vi "CLC_GEN3_L2_InPhaseCal_mW.vi"() -> ()   [LabVIEW 2023, in "Clover_Cell.lvlib"]
uses:
  Clover_Cell.lvlib
  lib/Anritsu Signal Analyzer Series/Anritsu Signal Analyzer Series.lvlib
  lib/ELTA/ELTA.lvlib
panel:
  in  "Daul_Ch_Phase_Sweep":bool
  in  "SweepSwitch?":u16(ring) items=["NoSweep(Single)", "Sweep"]
  in  "SweepMode":u16(ring) items=["Phase", "Gain"]
  in  "Method":u16(ring)=1 items=["dBm"=1, "mW"=2]
  in  "Polarity":u16(ring) items=["H", "V"]
  in  "VISA resource name":refnum<visa-resource-name>="TCPIP0::192.168.100.230::inst0::INSTR"
  in  "CenterFreq(GHz)":dbl=28.0
  in  "AvgTimes":i32=3
  in  "Single_Ch_Phase_Sweep":bool
  in  "TRXmode":u16(ring)=1 items=["Rx"=2, "Tx"=1]
  out "GainStep":i32=63
  out "PhaseStep":i32=63
  out "Channel":i32=63
  out "Total mW":dbl format="%.7f"
  out "Total dBm":dbl format="%.7f"
  out "Ref. mW":dbl format="%.7f"
  out "Ref. dBm":dbl format="%.7f"
  out "Main mW":dbl format="%.7f"
  out "Main dBm":dbl format="%.7f"
  out "Data":dbl[][](array[numeric])
  out "FileNAME_Single":string
  out "Spectrum Analyzer":dbl[](graph)
  out "CurrentData":dbl[](array[numeric])
  out "Duration":dbl
  out "TotalTime":dbl format="%.2f"
  out "StopTime":timestamp=timestamp(3663835912.033212 s since 1904-01-01)
  out "FileNAME_Dual":string
  out "StartTime":timestamp=timestamp(3663835741.875155 s since 1904-01-01)
  out "TX/RX":u16=1
  out "error out":errorcluster
  out "output cluster":T1={"address"="192.168.100.111", "remote port or service name"=5025, "timeout ms (60000)"=10000}
  out "Operating \nChannel(s)":bool[][](array[boolean])
  out "OK?":bool
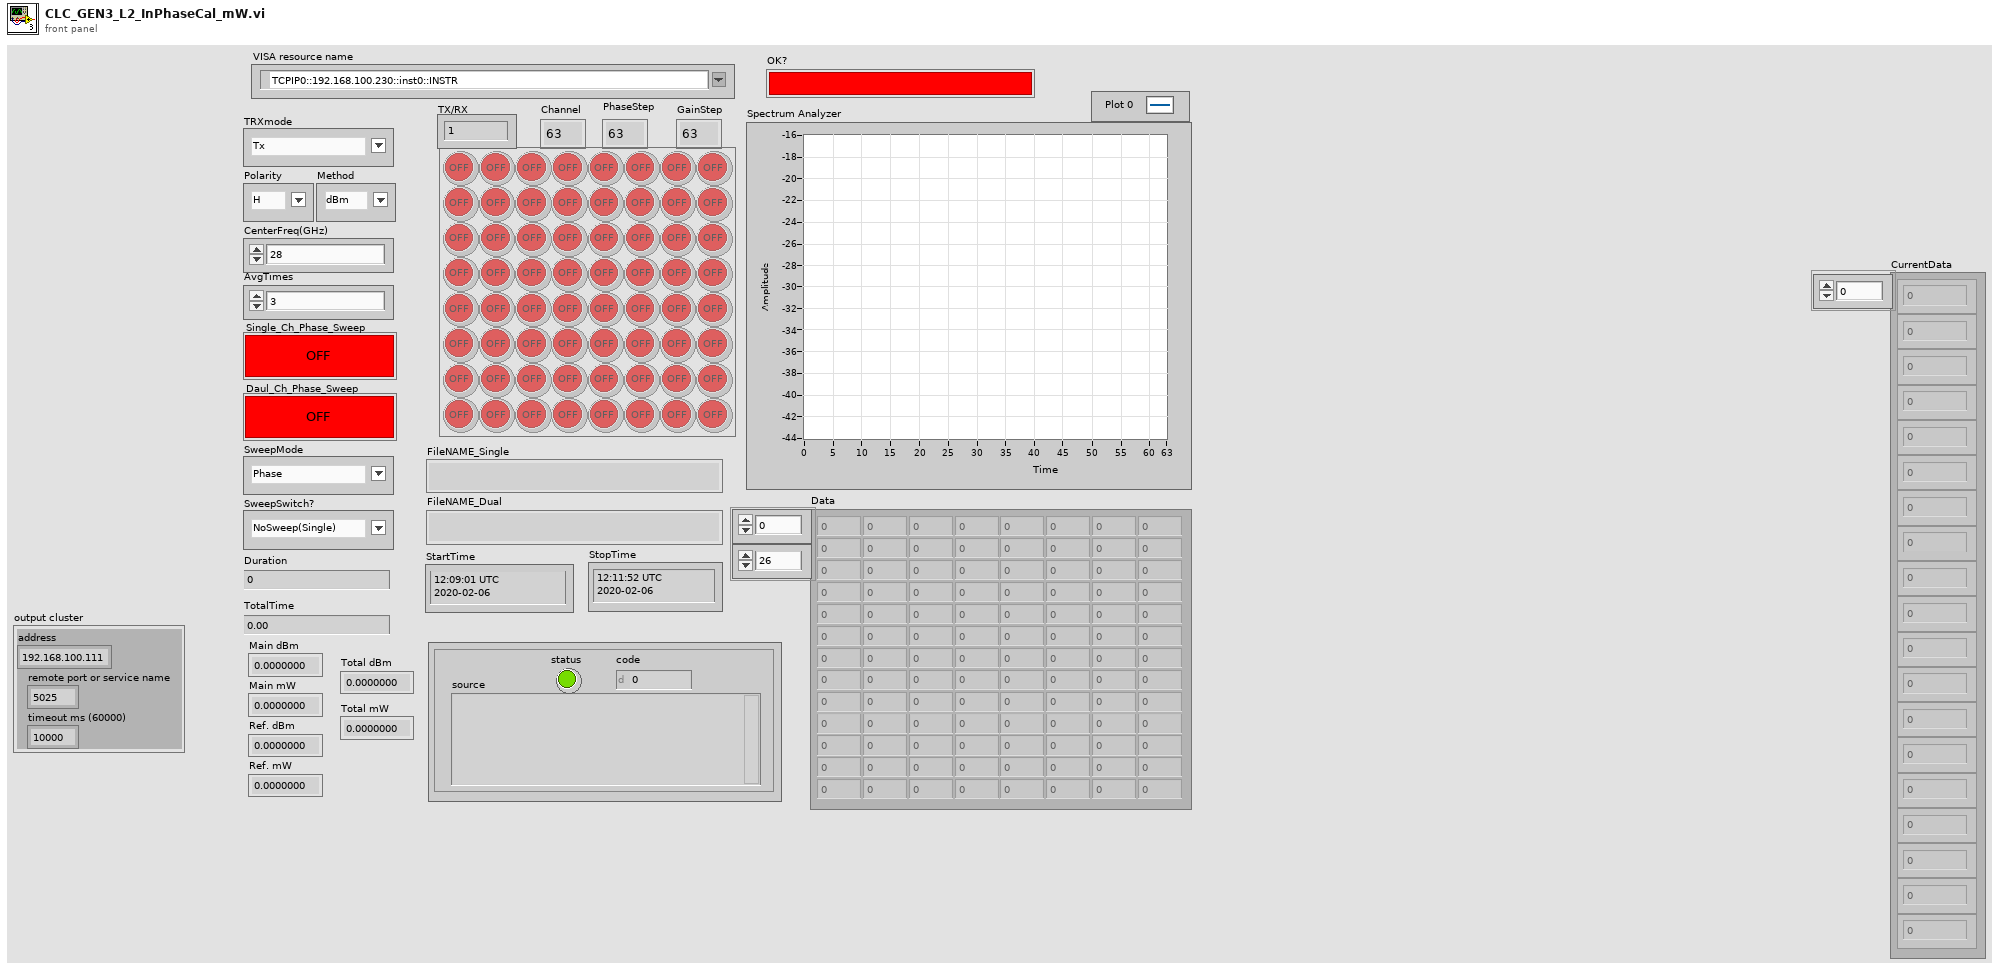
[diagram p1: front panel]
types:
  T1 = cluster{"address":string, "remote port or service name":u16, "timeout ms (60000)":i32}
  T2 = cluster{"Mode":u16, "Polarity":u16, "CH_ON/OFF":u16, "Channel":i32, "Gain":i32, "Phase":i32}
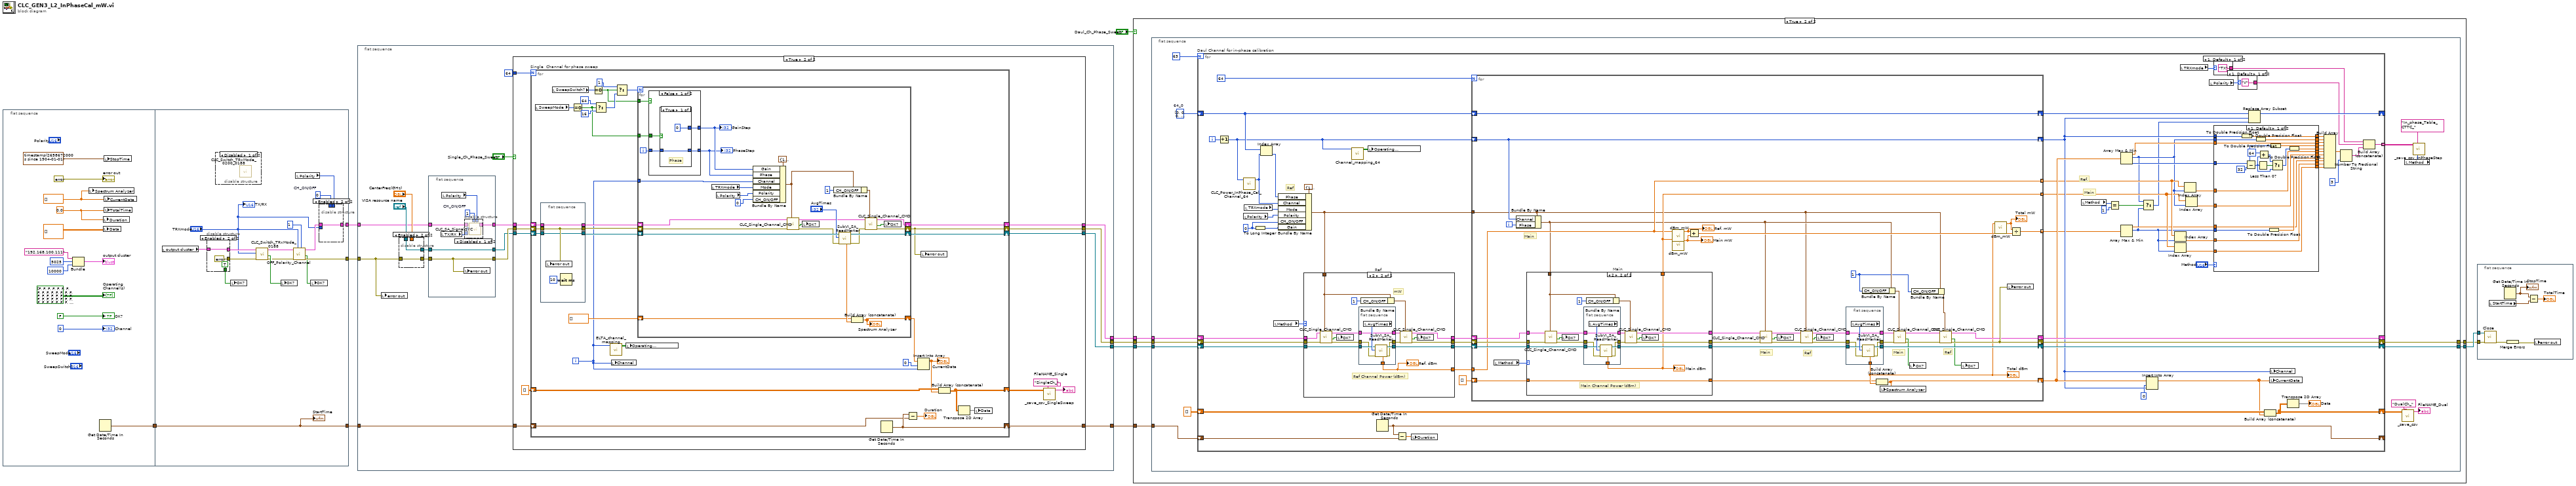
[diagram p0: block diagram]
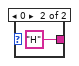
[diagram p3: hidden frame]
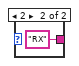
[diagram p4: hidden frame]
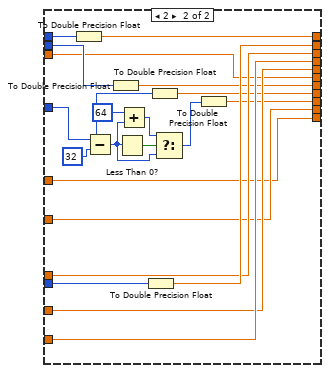
[diagram p5: hidden frame]
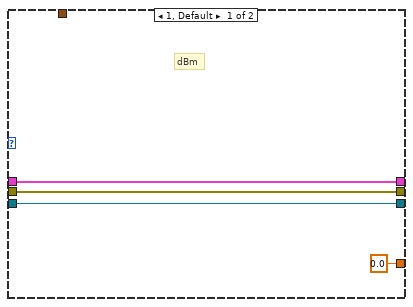
[diagram p6: hidden frame]
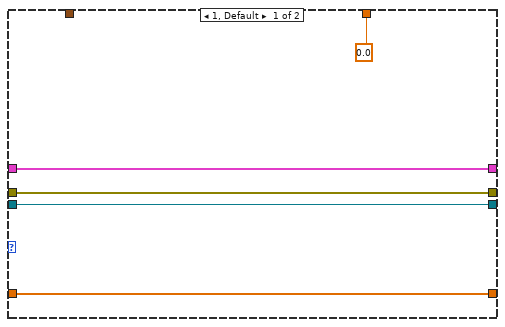
[diagram p7: hidden frame]
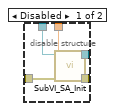
[diagram p8: hidden frame]
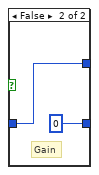
[diagram p10: hidden frame]
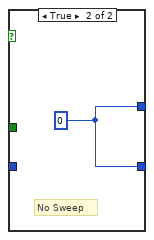
[diagram p11: hidden frame]
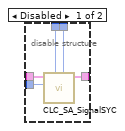
[diagram p14: hidden frame]
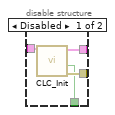
[diagram p15: hidden frame]
diagram:
  n1 = flat-sequence {
    tunnel: [w12] -> w11
    tunnel: w11 -> [w28]
    tunnel: [w31] -> w2
    tunnel: [w35] -> w3
    tunnel: [w28] -> w10
    frame #0 {
      w16 = dbl[] []
      w19 = 0.0 ("TotalTime")
      n2 = Bundle("address"="192.168.100.111", "remote port or service name"=u16 5025, "timeout ms (60000)"=10000) -> (→"output cluster":T1)  [unwired: 1 in]
      n3 = local write "Spectrum Analyzer"(w16) -> ()
      n4 = Get Date/Time In Seconds() -> (seconds since 1Jan1904=w12:timestamp)
      n5 = local write "Duration"(w19) -> ()
      n6 = local write "Data"(dbl[][] []) -> ()
      n7 = local write "StopTime"(timestamp(2658672000.001 s since 1904-01-01) ("StopTime")) -> ()
      n8 = local write "CurrentData"(w16) -> ()
      n9 = local write "TotalTime"(w19) -> ()
      "error out" <- errorcluster {"status"=FALSE, "code"=0, "source"=""} ("error out")
      "Operating \nChannel(s)" <- bool[][] [[FALSE, FALSE, FALSE, FALSE, FALSE, FALSE, FALSE, FALSE], [FALSE, FALSE, FALSE, FALSE, FALSE, FALSE, FALSE, FALSE], [FALSE, FALSE, FALSE, FALSE, FALSE, FALSE, FALSE, FALSE], [FALSE, FALSE, FALSE, FALSE, FALSE, FALSE, FALSE, FALSE], [FALSE, FALSE, FALSE, FALSE, FALSE, FALSE, FALSE, FALSE], [FALSE, FALSE, FALSE, FALSE, FALSE, FALSE, FALSE, FALSE], [FALSE, FALSE, FALSE, FALSE, FALSE, FALSE, FALSE, FALSE], [FALSE, FALSE, FALSE, FALSE, FALSE, FALSE, FALSE, FALSE]] ("Operating \nChannel(s)")
      "Channel" <- 0 ("Channel")
      "OK?" <- FALSE ("OK?")
    }
    frame #1 {
      w30 = u16 0  # CH_ON/OFF
      n10 = local read "output cluster"() -> (w40:T1)
      n11 = disable-structure shown="Enabled" {
        disable-tunnel: w40 -> [w50 w53]
        disable-tunnel: [w49 w53] -> w39
        disable-tunnel: [w48 errorcluster {"status"=FALSE, "code"=0, "source"=""} ("error in (no error)")] -> w37
        disable-tunnel: [w47 TRUE ("OK?")] -> w29
        frame Disabled {
          n12 = call "CLC_Init.vi"("TCPIPin"=w50) -> ("error out"=w48:errorcluster, "Status"=w47:bool, "TCPIPin 2"=w49:T1)  [unwired: 8 in]
        }
        frame Enabled {
        }
      }
      n13 = disable-structure shown="Disabled" {
        frame Disabled {
          n14 = call "CLC_Switch_TRxMode_0200_0188.vi"() -> ()  [unwired: 9 in, 3 out]
        }
        frame Enabled {
        }
      }
      n15 = local write "OK?"(w29) -> ()
      n16 = call "CLC_Switch_TRxMode_0188.vi"("error in (no error)"=w37, "Text Ring"="TRXmode", "TCPIPin"=w39) -> ("error out"=w36:errorcluster, "OK?"=w38:bool, "TCPIPin 2"=w34:T1)  [unwired: 6 in]
      n17 = local write "OK?"(w38) -> ()
      n18 = call "OFF_Polarity_Channel.vi"("CH_ON:0/OFF:1"=u16 1, "Mode"="TRXmode", "error in"=w36, "TCPIPin"=w34) -> ("error out"=w35:errorcluster, "OK?"=w33:bool, "TCPIPout"=w32:T1)  [unwired: 5 in]
      n19 = local read "Polarity"() -> (w26:u16)
      n20 = local write "OK?"(w33) -> ()
      n21 = disable-structure shown="Enabled" {
        disable-tunnel: w32 -> [w45 w46]
        disable-tunnel: [w44 w46] -> w31
        disable-tunnel: w30 -> [w43 _]
        disable-tunnel: w26 -> [w42 _]
        disable-tunnel: "TRXmode" -> [w41 _]
        frame Disabled {
          n22 = call "CLC_SA_SignalSYC.vi"("Polarity"=w42, "CH_ON/OFF"=w43, "Mode"=w41, "TCPIPin"=w45) -> ("TCPIPout"=w44:T1)  [unwired: 7 in]
        }
        frame Enabled {
        }
      }
      "StartTime" <- w28
      "TX/RX" <- "TRXmode"
    }
  }
  n23 = flat-sequence {
    tunnel: w10 -> [w67]
    tunnel: [w66] -> w9
    tunnel: [w65] -> w8
    tunnel: [w64] -> w7
    tunnel: [w63] -> w4
    tunnel: w3 -> [w61]
    tunnel: w2 -> [w58]
    frame #0 {
      n24 = local write "error out"(w61) -> ()
      n25 = disable-structure shown="Enabled" {
        disable-tunnel: "VISA resource name" -> [w74 w75]
        disable-tunnel: [w73 w76] -> w62
        disable-tunnel: w61 -> [w72 w76]
        disable-tunnel: "CenterFreq(GHz)" -> [w71 _]
        disable-tunnel: [w70 w75] -> w57
        frame Disabled {
          n26 = call "SubVI_SA_Init.vi"("error in (no error)"=w72, "CenterFreq(GHz) 2"=w71, "VISA resource name"=w74) -> ("error out 2"=w73:errorcluster, "VISA resource name out"=w70:refnum<visa-resource-name>)  [unwired: 6 in, 1 out]
        }
        frame Enabled {
        }
      }
      n27 = flat-sequence {
        tunnel: w62 -> [w171]
        tunnel: [w171] -> w59
        tunnel: w58 -> [w169]
        tunnel: w57 -> [w170]
        tunnel: [w170] -> w56
        tunnel: [w168] -> w55
        frame #0 {
          w167 = u16 1  # CH_ON/OFF
          n28 = local read "TX/RX"() -> (w165:u16)
          n29 = local read "Polarity"() -> (w166:u16)
          n30 = local write "error out"(w171) -> ()
          n31 = disable-structure shown="Disabled" {
            disable-tunnel: w169 -> [w176 w177]
            disable-tunnel: [w175 w177] -> w168
            disable-tunnel: w167 -> [w174 _]
            disable-tunnel: w166 -> [w173 _]
            disable-tunnel: w165 -> [w172 _]
            frame Disabled {
              n32 = call "CLC_SA_SignalSYC.vi"("Polarity"=w173, "CH_ON/OFF"=w174, "Mode"=w172, "TCPIPin"=w176) -> ("TCPIPout"=w175:T1)  [unwired: 7 in]
            }
            frame Enabled {
            }
          }
        }
      }
      n33 = case shown="True" "Single_Ch_Phase_Sweep" {
        tunnel: 64 -> [_ w93]
        tunnel: w67 -> [w77 w92]
        tunnel: [w78 w91] -> w66
        tunnel: [w79 w90] -> w65
        tunnel: [w80 w89] -> w64
        tunnel: [w77 w88] -> w63
        tunnel: w59 -> [w79 w87]
        tunnel: w56 -> [w78 w86]
        tunnel: w55 -> [w80 w85]
        frame False {
        }
        frame True {
          n34 = for "Single  Channel for phase sweep" {
            N: w93 -> [_]
            shift-right: [w123] -> w89
            shift-left: w85 -> [w109]
            shift-right: [w118] -> w90
            shift-left: w87 -> [w111]
            shift-right: [w122] -> w91
            shift-left: w86 -> [w108]
            shift-right: [w116] -> w82
            shift-left: dbl[][] [] -> [w117]
            shift-right: [w120] -> w88
            shift-left: w92 -> [w119]
            i -> [w94]
            n35 = local read "SweepMode"() -> (w103:u16)
            n36 = flat-sequence {
              tunnel: [w125] -> w107
              tunnel: w111 -> [w126]
              tunnel: [w126] -> w110
              tunnel: w109 -> [w125]
              tunnel: w108 -> [w124]
              tunnel: [w124] -> w106
              frame #0 {
                n37 = local write "error out"(w126) -> ()
                n38 = Wait (ms)(milliseconds to wait=u32 10) -> ()  [unwired: 1 out]
              }
            }
            n39 = local read "SweepSwitch?"() -> (w102:u16)
            n40 = Equal To 0?(x=w103) -> (x = 0?=w95:bool)
            n41 = Equal To 0?(x=w102) -> (x = 0?=w96:bool)
            n42 = Select(t=64, s=w95, f=16) -> (s? t:f=w97:i32)
            n43 = call "ELTA_channel_mapping.vi"("Ch_1_ref"=w94) -> ("Operating \nChannel(s)"=w104:bool[][])  [unwired: 10 in]
            n44 = local write "Channel"(w94) -> ()
            n45 = Select(t=1, s=w96, f=w97) -> (s? t:f=w100:i32)
            n46 = local write "Operating \nChannel(s)"(w104) -> ()
            n47 = for {
              N: w100 -> [_]
              shift-right: [w137] -> w123
              shift-left: w107 -> [w147]
              shift-right: [w139] -> w118
              shift-left: w110 -> [w149]
              shift-right: [w154] -> w122
              shift-left: w106 -> [w155]
              shift-right: [w150] -> w115
              shift-left: dbl[] [] -> [w151]
              tunnel: w94 -> [w144]
              tunnel: w96 -> [w132]
              tunnel: w95 -> [w129]
              i -> [w128]
              n48 = case shown="False" w132 {
                tunnel: [w156 w164] -> w131
                tunnel: [w157 w164] -> w130
                tunnel: w129 -> [w159 _]
                tunnel: w128 -> [w158 _]
                frame False {
                  n49 = case shown="True" w159 {
                    tunnel: w158 -> [w161 w162]
                    tunnel: [w161 0] -> w157
                    tunnel: [0 w162] -> w156
                    frame True {
                      # "Phase"
                    }
                    frame False {
                      # "Gain"
                    }
                  }
                }
                frame True {
                  w164 = 0
                  # "No Sweep"
                }
              }
              "PhaseStep" <- w130
              "GainStep" <- w131
              n50 = local read "TRXmode"() -> (w143:u16)
              n51 = local read "Polarity"() -> (w142:u16)
              n52 = Bundle By Name(cluster=T2 {"Mode"=1, "Polarity"=1, "CH_ON/OFF"=1, "Channel"=0, "Gain"=0, "Phase"=0} ("Channel params"), "Gain"=w131, "Phase"=w130, "Channel"=w144, "Mode"=w143, "Polarity"=w142, "CH_ON/OFF"=u16 0) -> (w136:T2)
              n53 = call "CLC_Single_Channel_CMD.vi"("Channel params"=w136, "error in"=w149, "TCPIPin"=w147) -> ("error out"=w148:errorcluster, "OK?"=w145:bool, "TCPIPout"=w138:T1)  [unwired: 6 in]
              n54 = local write "OK?"(w145) -> ()
              n55 = Bundle By Name(cluster=w136, "CH_ON/OFF"=u16 1) -> (w134:T2)
              n56 = call "SubVI_SA_ReadMarker.vi"("error in (no error)"=w148, "AvgTimes"="AvgTimes", "VISA resource name"=w155) -> ("error out"=w140:errorcluster, "VISA resource name out"=w154:refnum<visa-resource-name>, "Marker Power"=w152:dbl)  [unwired: 5 in, 1 out]
              n57 = Build Array (concatenate)(w151, w152) -> (w150:dbl[])
              "Spectrum Analyzer" <- w150
              n58 = call "CLC_Single_Channel_CMD.vi"("Channel params"=w134, "error in"=w140, "TCPIPin"=w138) -> ("error out"=w139:errorcluster, "OK?"=w133:bool, "TCPIPout"=w137:T1)  [unwired: 6 in]
              n59 = local write "OK?"(w133) -> ()
            }
            n60 = Get Date/Time In Seconds() -> (seconds since 1Jan1904=w120:timestamp)
            n61 = Subtract(x=w120, y=w119) -> (x-y=→"Duration":dbl)
            n62 = Insert Into Array(array=w115, index=0, new element=w94) -> (w113:dbl[])
            "CurrentData" <- w113
            n63 = local write "error out"(w118) -> ()
            n64 = Build Array (concatenate)(w117, w113) -> (w116:dbl[][])
            n65 = Transpose 2D Array(2D array=w116) -> (transposed array=w105:dbl[][])
            n66 = local write "Data"(w105) -> ()
          }
          n67 = call "_save_csv_SingleSweep.vi"("delimiter (\\t)"="SingleCh_" ("delimiter (\\t)"), "Data"=w82) -> ("FileName"=→"FileNAME_Single":string)  [unwired: 9 in]
        }
      }
    }
  }
  n68 = case shown="True" "Daul_Ch_Phase_Sweep" {
    tunnel: w9 -> [w179 w185]
    tunnel: w8 -> [w178 w184]
    tunnel: w7 -> [_ w183]
    tunnel: [w179 w182] -> w6
    tunnel: [w178 w181] -> w5
    tunnel: w4 -> [_ w180]
    frame False {
    }
    frame True {
      n69 = flat-sequence {
        tunnel: w185 -> [w199]
        tunnel: w184 -> [w198]
        tunnel: w183 -> [w197]
        tunnel: [w196] -> w182
        tunnel: [w195] -> w181
        tunnel: w180 -> [w194]
        frame #0 {
          w192 = i32[] [0, 0, 0, 0, 0, 0, 0, 0, 0, 0, 0, 0, 0, 0, 0, 0, 0, 0, 0, 0, 0, 0, 0, 0, 0, 0, 0, 0, 0, 0, 0, 0, 0, 0, 0, 0, 0, 0, 0, 0, 0, 0, 0, 0, 0, 0, 0, 0, 0, 0, 0, 0, 0, 0, 0, 0, 0, 0, 0, 0, 0, 0, 0, 0]  # 64_0
          n70 = for "Daul Channel for in-phase calibration" {
            N: 63 -> [_]
            shift-right: [w273] -> _
            shift-left: w197 -> [w237]
            shift-right: [w270] -> w195
            shift-left: w198 -> [w241]
            shift-right: [w271] -> w196
            shift-left: w199 -> [w239]
            shift-right: [w265] -> w187
            shift-left: dbl[][] [] -> [w266]
            shift-right: [w269] -> _
            shift-left: w194 -> [w268]
            shift-right: [w259] -> _
            shift-left: w192 -> [w234]
            tunnel: [w203] -> w188 mode=indexing
            i -> [w202]
            w243 = u16 0 ("CH_ON/OFF")
            # "Main"
            # "Ref."
            # "Ref"
            n71 = Increment(x=w202) -> (x+1=w201:i32)
            n72 = call "CLC_Power_InPhase_Cal_Channel_64.vi"("Channel IN"=w201) -> ("Ref_Channel"=w230:i32)  [unwired: 8 in, 2 out]
            n73 = local read "Polarity"() -> (w244:u16)
            n74 = local read "TRXmode"() -> (w245:u16)
            n75 = To Long Integer(number=w243) -> (32bit integer=w242:i32)
            n76 = Index Array(array=w234, index=w230) -> (element=w233:i32)
            n77 = local read "Method"() -> (w231:u16)
            n78 = Bundle By Name(cluster=T2 {"Mode"=1, "Polarity"=1, "CH_ON/OFF"=1, "Channel"=0, "Gain"=0, "Phase"=0} ("Channel params"), "Phase"=w233, "Channel"=w230, "Mode"=w245, "Polarity"=w244, "CH_ON/OFF"=w243, "Gain"=w242) -> (w232:T2)
            n79 = case "Ref" shown="2" w231 {
              tunnel: w241 -> [w322 w331]
              tunnel: [w322 w330] -> w240
              tunnel: w239 -> [w321 w329]
              tunnel: [w321 w328] -> w238
              tunnel: w237 -> [w323 w327]
              tunnel: [w323 w326] -> w236
              tunnel: [0.0 ("Marker Response") w325] -> w235
              tunnel: w232 -> [_ w324]
              frame 1, Default {
                # "dBm"
              }
              frame 2 {
                # "mW"
                # "Ref Channel Power (dBm)"
                n80 = call "CLC_Single_Channel_CMD.vi"("Channel params"=w324, "error in"=w331, "TCPIPin"=w327) -> ("error out"=w338:errorcluster, "OK?"=w339:bool, "TCPIPout"=w337:T1)  [unwired: 6 in]
                n81 = local write "OK?"(w339) -> ()
                n82 = flat-sequence {
                  tunnel: [w346] -> w328
                  tunnel: [w344] -> w325
                  tunnel: w329 -> [w343]
                  tunnel: w338 -> [w342]
                  tunnel: [w341] -> w333
                  tunnel: w337 -> [w341]
                  tunnel: [w340] -> w334
                  frame #0 {
                    n83 = local read "AvgTimes"() -> (w345:i32)
                    n84 = call "SubVI_SA_ReadMarker.vi"("error in (no error)"=w342, "AvgTimes"=w345, "VISA resource name"=w343) -> ("error out"=w340:errorcluster, "VISA resource name out"=w346:refnum<visa-resource-name>, "Marker Power"=w344:dbl)  [unwired: 5 in, 1 out]
                  }
                }
                n85 = Bundle By Name(cluster=w324, "CH_ON/OFF"=u16 1) -> (w335:T2)
                n86 = call "CLC_Single_Channel_CMD.vi"("Channel params"=w335, "error in"=w334, "TCPIPin"=w333) -> ("error out"=w330:errorcluster, "OK?"=w336:bool, "TCPIPout"=w326:T1)  [unwired: 6 in]
                n87 = local write "OK?"(w336) -> ()
                "Ref. dBm" <- w325
              }
            }
            n88 = call "Channel_mapping_64.vi"("Channel IN"=w201) -> ("Operating \nChannel(s)"=w247:bool[][])  [unwired: 10 in]
            n89 = local write "Operating \nChannel(s)"(w247) -> ()
            n90 = Get Date/Time In Seconds() -> (seconds since 1Jan1904=w269:timestamp)
            n91 = Subtract(x=w269, y=w268) -> (x-y=w267:dbl)
            n92 = local write "Duration"(w267) -> ()
            n93 = for {
              N: 64 -> [_]
              shift-right: [w372] -> w273
              shift-left: w236 -> [w355]
              shift-right: [w376] -> w270
              shift-left: w240 -> [w368]
              shift-right: [w387] -> w271
              shift-left: w238 -> [w367]
              shift-right: [w370] -> w260
              shift-left: dbl[] [] -> [w357]
              shift-right: [w381] -> w258
              shift-left: w234 -> [w381]
              shift-right: [w350] -> w257
              shift-left: w201 -> [w350]
              tunnel: [w354] -> w250 mode=indexing
              tunnel: [w361] -> w249 mode=indexing
              tunnel: [w362] -> w256 mode=indexing
              tunnel: w232 -> [w348]
              tunnel: w235 -> [w354]
              i -> [w351]
              w347 = u16 1 ("CH_ON/OFF")
              # "Main"
              # "Ref"
              # "Main"
              # "Ref"
              # "Main"
              n94 = local read "Method"() -> (w358:u16)
              n95 = Bundle By Name(cluster=w348, "Channel"=w350, "Phase"=w351) -> (w349:T2)
              n96 = case "Main" shown="2" w358 {
                tunnel: w368 -> [w390 w396]
                tunnel: w355 -> [w391 w397]
                tunnel: w367 -> [w389 w395]
                tunnel: [w391 w401] -> w366
                tunnel: [w390 w400] -> w365
                tunnel: [w389 w399] -> w364
                tunnel: w349 -> [_ w398]
                tunnel: [0.0 ("Marker Response") w393] -> w361
                tunnel: w357 -> [w388 w394]
                tunnel: [w388 w394] -> w356
                frame 1, Default {
                }
                frame 2 {
                  # "Main Channel Power (dBm)"
                  n97 = call "CLC_Single_Channel_CMD.vi"("Channel params"=w398, "error in"=w396, "TCPIPin"=w397) -> ("error out"=w403:errorcluster, "OK?"=w402:bool, "TCPIPout"=w404:T1)  [unwired: 6 in]
                  n98 = local write "OK?"(w402) -> ()
                  n99 = flat-sequence {
                    tunnel: [w416] -> w399
                    tunnel: [w414] -> w393
                    tunnel: w395 -> [w413]
                    tunnel: w403 -> [w412]
                    tunnel: [w411] -> w409
                    tunnel: w404 -> [w411]
                    tunnel: [w410] -> w408
                    frame #0 {
                      n100 = local read "AvgTimes"() -> (w415:i32)
                      n101 = call "SubVI_SA_ReadMarker.vi"("error in (no error)"=w412, "AvgTimes"=w415, "VISA resource name"=w413) -> ("error out"=w410:errorcluster, "VISA resource name out"=w416:refnum<visa-resource-name>, "Marker Power"=w414:dbl)  [unwired: 5 in, 1 out]
                    }
                  }
                  n102 = Bundle By Name(cluster=w398, "CH_ON/OFF"=u16 1) -> (w407:T2)
                  n103 = call "CLC_Single_Channel_CMD.vi"("Channel params"=w407, "error in"=w408, "TCPIPin"=w409) -> ("error out"=w400:errorcluster, "OK?"=w405:bool, "TCPIPout"=w401:T1)  [unwired: 6 in]
                  n104 = local write "OK?"(w405) -> ()
                  "Main dBm" <- w393
                }
              }
              n105 = call "dBm_mW.vi"("dBm"=w354) -> ("mW"=w353:dbl)  [unwired: 10 in]
              "Ref. mW" <- w353
              n106 = call "dBm_mW.vi"("dBm"=w361) -> ("mW"=w352:dbl)  [unwired: 10 in]
              "Main mW" <- w352
              n107 = Add(x=w353, y=w352) -> (x+y=w363:dbl)
              n108 = call "CLC_Single_Channel_CMD.vi"("Channel params"=w349, "error in"=w365, "TCPIPin"=w366) -> ("error out"=w385:errorcluster, "OK?"=w384:bool, "TCPIPout"=w386:T1)  [unwired: 6 in]
              n109 = local write "OK?"(w384) -> ()
              n110 = call "CLC_Single_Channel_CMD.vi"("Channel params"=w348, "error in"=w385, "TCPIPin"=w386) -> ("error out"=w382:errorcluster, "OK?"=w383:bool, "TCPIPout"=w380:T1)  [unwired: 6 in]
              n111 = local write "OK?"(w383) -> ()
              n112 = flat-sequence {
                tunnel: [w423] -> w387
                tunnel: [w421] -> w360
                tunnel: w364 -> [w420]
                tunnel: w382 -> [w419]
                tunnel: [w418] -> w379
                tunnel: w380 -> [w418]
                tunnel: [w417] -> w369
                frame #0 {
                  n113 = local read "AvgTimes"() -> (w422:i32)
                  n114 = call "SubVI_SA_ReadMarker.vi"("error in (no error)"=w419, "AvgTimes"=w422, "VISA resource name"=w420) -> ("error out"=w417:errorcluster, "VISA resource name out"=w423:refnum<visa-resource-name>, "Marker Power"=w421:dbl)  [unwired: 5 in, 1 out]
                }
              }
              n115 = Bundle By Name(cluster=w349, "CH_ON/OFF"=w347) -> (w371:T2)
              n116 = Build Array (concatenate)(w356, w360) -> (w370:dbl[])
              n117 = local write "Spectrum Analyzer"(w370) -> ()
              n118 = call "CLC_Single_Channel_CMD.vi"("Channel params"=w371, "error in"=w369, "TCPIPin"=w379) -> ("error out"=w377:errorcluster, "OK?"=w378:bool, "TCPIPout"=w375:T1)  [unwired: 6 in]
              n119 = local write "OK?"(w378) -> ()
              n120 = Bundle By Name(cluster=w348, "CH_ON/OFF"=w347) -> (w374:T2)
              n121 = call "CLC_Single_Channel_CMD.vi"("Channel params"=w374, "error in"=w377, "TCPIPin"=w375) -> ("error out"=w376:errorcluster, "OK?"=w373:bool, "TCPIPout"=w372:T1)  [unwired: 6 in]
              n122 = local write "OK?"(w373) -> ()
              n123 = call "dBm_mW.vi"("dBm"=w360) -> ("mW"=w359:dbl)  [unwired: 10 in]
              "Total mW" <- w359
              n124 = local write "error out"(w376) -> ()
              n125 = Divide(x=w359, y=w363) -> (x/y=w362:dbl)
              "Total dBm" <- w360
            }
            n126 = local read "Method"() -> (w217:u16)
            n127 = Equal?(x=w217, y=u16 1) -> (x = y?=w215:bool)
            n128 = Array Max & Min(array=w260) -> (max value=w227:dbl, max index (indices)=w214:i32, min index (indices)=w248:i32)  [unwired: 1 out]
            n129 = Array Max & Min(array=w256) -> (max value=w221:dbl, max index (indices)=w213:i32)  [unwired: 2 out]
            n130 = Select(t=w214, s=w215, f=w213) -> (s? t:f=w212:i32)
            n131 = Insert Into Array(array=w260, index=0, new element=w257) -> (w261:dbl[])
            n132 = Index Array(array=w250, index=w213) -> (element=w220:dbl)
            n133 = Index Array(array=w249, index=w213) -> (element=w219:dbl)
            n134 = local read "TRXmode"() -> (w208:u16)
            n135 = Index Array(array=w250, index=w214) -> (element=w225:dbl)
            n136 = Index Array(array=w249, index=w214) -> (element=w224:dbl)
            n137 = local read "Polarity"() -> (w207:u16)
            n138 = case shown="1, Default" w208 {
              tunnel: ["TX" "RX"] -> w204
              frame 1, Default {
              }
              frame 2 {
              }
            }
            n139 = case shown="1, Default" "Method" {
              tunnel: w257 -> [w292 w313]
              tunnel: [w278 w307] -> w255
              tunnel: [w291 w306] -> w254
              tunnel: [w290 w305] -> w253
              tunnel: [w289 w309] -> w252
              tunnel: [w288 w302] -> w251
              tunnel: w248 -> [w287 w312]
              tunnel: w213 -> [w286 w311]
              tunnel: w214 -> [w285 w310]
              tunnel: w227 -> [w278 w304]
              tunnel: [w279 w308] -> w228
              tunnel: [w284 w304] -> w226
              tunnel: w225 -> [w284 w299]
              tunnel: w224 -> [w283 w300]
              tunnel: [w283 w303] -> w223
              tunnel: [w282 w301] -> w222
              tunnel: w221 -> [w282 w307]
              tunnel: w220 -> [w281 w305]
              tunnel: w219 -> [w280 w306]
              tunnel: [w280 w299] -> w218
              tunnel: [w281 w300] -> w211
              frame 1, Default {
                n140 = To Double Precision Float(number=w292) -> (double precision float=w289:dbl)
                n141 = Subtract(x=w287, y=32) -> (x-y=w294:i32)
                n142 = To Double Precision Float(number=w285) -> (double precision float=w279:dbl)
                n143 = Less Than 0?(x=w294) -> (x < 0?=w297:bool)
                n144 = Add(x=64, y=w294) -> (x+y=w295:i32)
                n145 = To Double Precision Float(number=w286) -> (double precision float=w288:dbl)
                n146 = To Double Precision Float(number=w287) -> (double precision float=w291:dbl)
                n147 = Select(t=w295, s=w297, f=w294) -> (s? t:f=w293:i32)
                n148 = To Double Precision Float(number=w293) -> (double precision float=w290:dbl)
              }
              frame 2 {
                n149 = To Double Precision Float(number=w313) -> (double precision float=w309:dbl)
                n150 = Subtract(x=w312, y=32) -> (x-y=w315:i32)
                n151 = To Double Precision Float(number=w310) -> (double precision float=w303:dbl)
                n152 = Less Than 0?(x=w315) -> (x < 0?=w318:bool)
                n153 = Add(x=64, y=w315) -> (x+y=w316:i32)
                n154 = To Double Precision Float(number=w311) -> (double precision float=w308:dbl)
                n155 = To Double Precision Float(number=w312) -> (double precision float=w302:dbl)
                n156 = Select(t=w316, s=w318, f=w315) -> (s? t:f=w314:i32)
                n157 = To Double Precision Float(number=w314) -> (double precision float=w301:dbl)
              }
            }
            n158 = case shown="1, Default" w207 {
              tunnel: ["V" "H"] -> w205
              frame 1, Default {
              }
              frame 0 {
              }
            }
            n159 = Replace Array Subset(array=w258, new element=w212, index=w257) -> (w259:i32[])
            n160 = Build Array (concatenate)(w266, w261) -> (w265:dbl[][])
            n161 = local write "CurrentData"(w261) -> ()
            n162 = local write "Channel"(w257) -> ()
            n163 = Transpose 2D Array(2D array=w265) -> (transposed array=→"Data":dbl[][])
            n164 = Build Array(w252, w228, w255, w254, w253, w226, w223, w251, w222, w211, w218) -> (w209:dbl[])
            n165 = Number To Fractional String(number=w209, precision (6)=i16 3) -> (F-format string=w206:string[])  [unwired: 2 in]
            n166 = Build Array (concatenate)(w204, w205, w206) -> (w203:string[])
          }
          n167 = call "_save_csv.vi"("delimiter (\\t)"="DualCh_" ("delimiter (\\t)"), "Data"=w187) -> ("FileName"=→"FileNAME_Dual":string)  [unwired: 9 in]
          n168 = local read "Method"() -> (w186:u16)
          n169 = call "_save_csv_InPhaseStep.vi"("Method"=w186, "delimiter (\\t)"="In_phase_Table_CTTC_" ("delimiter (\\t)"), "dataInput"=w188) -> ()  [unwired: 8 in, 1 out]
        }
      }
    }
  }
  n170 = flat-sequence {
    tunnel: w6 -> [w429]
    tunnel: w5 -> [w428]
    frame #0 {
      n171 = call "Close.vi"("error in (no error)"=w428, "VISA resource name"=w429) -> ("error out"=w430:errorcluster)  [unwired: 9 in]
      n172 = local read "StartTime"() -> (w424:timestamp)
      n173 = Get Date/Time In Seconds() -> (seconds since 1Jan1904=w425:timestamp)
      "StopTime" <- w425
      n174 = Merge Errors(w430) -> (w427:errorcluster)
      n175 = Subtract(x=w425, y=w424) -> (x-y=→"TotalTime":dbl)
      n176 = local write "error out"(w427) -> ()
    }
  }
